vi "send command to printer.vi"(8 "error in (no error)":errorcluster, 10 "command to be sent":string, 11 "Domino Laser module Class in":refnum<class "Domino Laser module Class.lvclass">) -> (0 "error out":errorcluster, 1 "Command Excuted succeddfully?":bool, 2 "Recived message":string, 3 "Domino Laser module Class out":refnum<class "Domino Laser module Class.lvclass">)   [LabVIEW 2024, in "Domino LM.lvlib" / "Domino Laser module Class.lvclass"]
uses:
  CTRLS/Domino Laser module Class.lvclass
  CTRLS/Domino Laser module Class.lvclass/Domino Laser module Class.ctl
panel:
  out "sent":string[](array[string])
  out "Recived":string[](array[string])
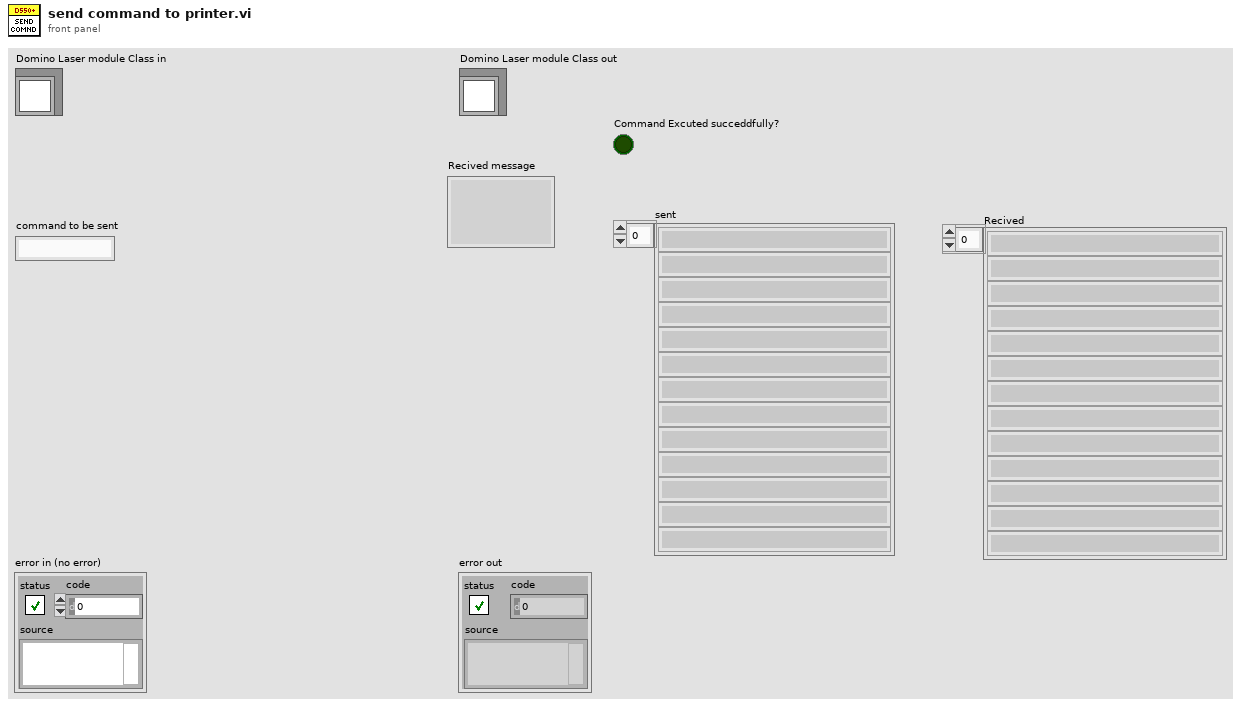
[diagram p1: front panel]
types:
  T1 = enum16{"Standard", "Buffered", "CRLF", "Immediate"}
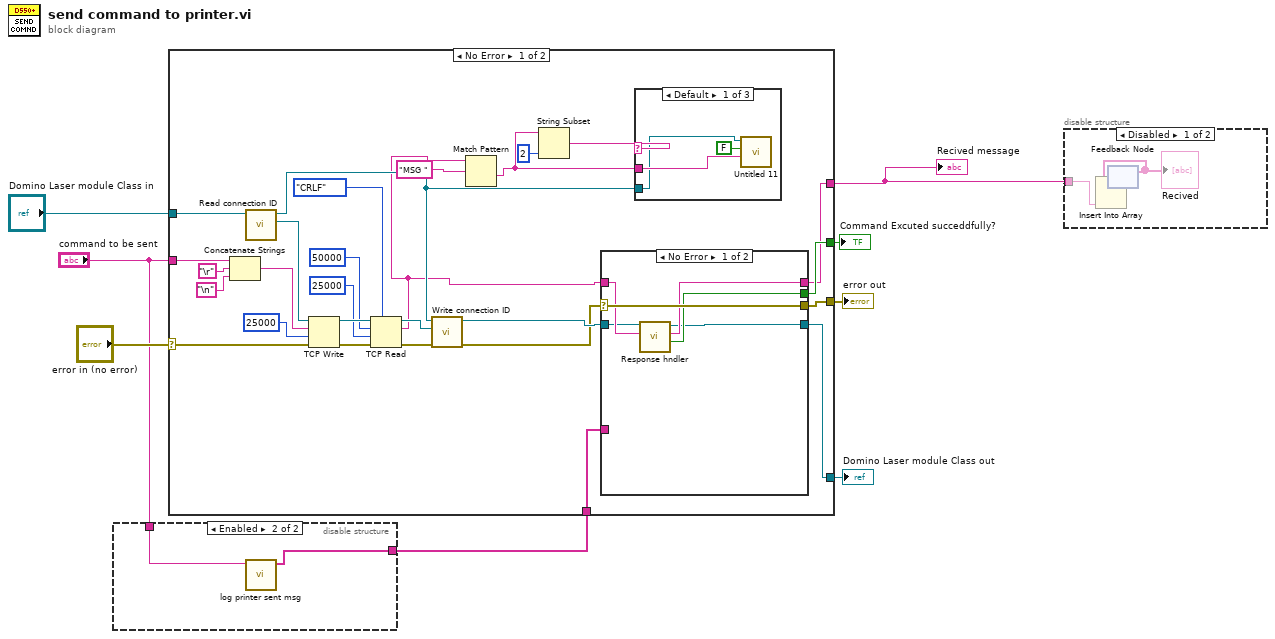
[diagram p0: block diagram]
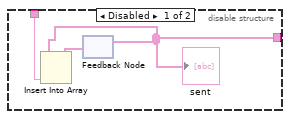
[diagram p3: hidden frame]
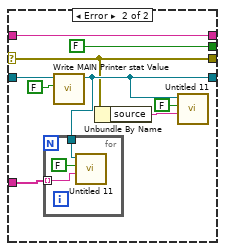
[diagram p4: hidden frame]
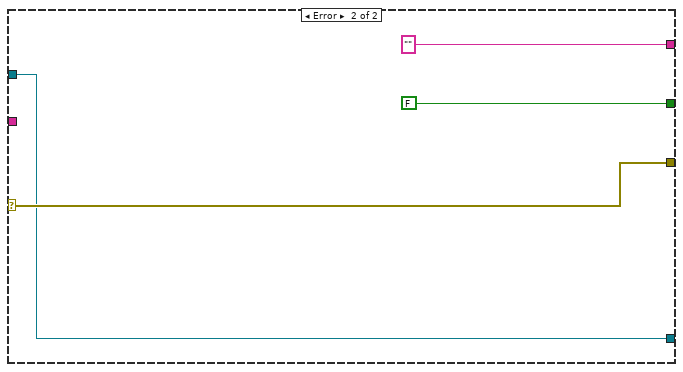
[diagram p7: hidden frame]
diagram:
  n1 = disable-structure shown="Enabled" {
    disable-tunnel: "command to be sent" -> [w10 w13]
    disable-tunnel: [w9 w12] -> w1
    frame Disabled {
      n2 = feedback #1() -> (w9:string[])  [unwired: 1 in]
      "sent" <- w9
      n3 = Insert Into Array(array=w9, new element=w10) -> (w11:string[])  [unwired: 1 in]
      n4 = feedback-in #1(w11) -> ()
    }
    frame Enabled {
      n5 = call "log printer sent msg.vi"("new element/subarray"=w13) -> ("sent 2"=w12:string[])  [unwired: 9 in, 1 out]
    }
  }
  n6 = case shown="No Error" "error in (no error)" {
    selector: "error in (no error)" -> [w28 w66]
    tunnel: [w17 w66] -> w7
    tunnel: [w16 w65] -> w5
    tunnel: "Domino Laser module Class in" -> [w27 w65]
    tunnel: [w15 "" ("data out")] -> w3
    tunnel: "command to be sent" -> [w29 _]
    tunnel: [w18 FALSE ("Command Excuted succeddfully?")] -> w4
    tunnel: w1 -> [w14 _]
    frame No Error {
      n7 = Concatenate Strings(w29, "\r", "\n") -> (w38:string)
      n8 = call "Read connection ID.vi"("Domino Laser module Class in"=w27) -> ("connection ID"=w39:refnum<k5>, "Domino Laser module Class out"=w22:refnum<class "Domino Laser module Class.lvclass">)  [unwired: 8 in, 1 out]
      n9 = TCP Write(connection ID=w39, data in=w38, error in (no error)=w28, 9:25000 ("timeout ms (25000)")) -> (connection ID out=w35:refnum<k5>, error out=w36:errorcluster)  [unwired: 1 out]
      n10 = TCP Read(connection ID=w35, bytes to read=50000 ("timeout ms (25000)"), error in (no error)=w36, 7:T1."CRLF" ("mode (standard)"), 9:25000 ("timeout ms (25000)")) -> (connection ID out=w33:refnum<k5>, data out=w19:string, error out=w32:errorcluster)
      n11 = call "Write connection ID.vi"("error in (no error)"=w32, "connection ID"=w33, "Domino Laser module Class in"=w22) -> ("error out"=w20:errorcluster, "Domino Laser module Class out"=w21:refnum<class "Domino Laser module Class.lvclass">)  [unwired: 7 in]
      n12 = Match Pattern(string=w19, regular expression="MSG ") -> (after substring=w25:string)  [unwired: 1 in, 3 out]
      n13 = String Subset(string=w25, length (rest)=2 ("length (rest)")) -> (substring=w23:string)  [unwired: 1 in]
      n14 = case shown="No Error" w20 {
        selector: w20 -> [w47 w51]
        tunnel: w21 -> [w43 w55]
        tunnel: [w42 w52] -> w16
        tunnel: w19 -> [w44 w54]
        tunnel: [w47 w51] -> w17
        tunnel: [w46 w54] -> w15
        tunnel: [w45 FALSE ("Command Excuted succeddfully?")] -> w18
        tunnel: w14 -> [_ w48]
        frame No Error {
          n15 = call "Response hndler.vi"("Recived MSG"=w44, "Domino LM.lvlib:Domino Laser module Class.lvclass"=w43) -> ("Command Excuted successfully?"=w45:bool, "printer response"=w46:string, "Domino LM.lvlib:Domino Laser module Class.lvclass 2"=w42:refnum<class "Domino Laser module Class.lvclass">)  [unwired: 7 in]
        }
        frame Error {
          n16 = call "Write MAIN Printer stat Value.vi"("Printer MIAN status"=FALSE ("Printer status"), "Domino Laser module Class in"=w55) -> ("Domino Laser module Class out"=w52:refnum<class "Domino Laser module Class.lvclass">)  [unwired: 8 in, 1 out]
          n17 = for {
            tunnel: w52 -> [w59]
            tunnel: w48 -> [w57] mode=indexing
            n18 = call "Untitled 11.vi"("MSG"=w57, "MSG Status"=FALSE, "Domino Laser module Class in"=w59) -> ()  [unwired: 7 in, 2 out]
          }
          n19 = Unbundle By Name(w51) -> ("source"=w50:string)
          n20 = call "Untitled 11.vi"("MSG"=w50, "MSG Status"=FALSE, "Domino Laser module Class in"=w52) -> ()  [unwired: 7 in, 2 out]
        }
      }
      n21 = case shown="Default" w23 {
        tunnel: w25 -> [w62 _ _]
        tunnel: w22 -> [w61 _ _]
        frame Default {
          n22 = call "Untitled 11.vi"("MSG"=w62, "MSG Status"=FALSE, "Domino Laser module Class in"=w61) -> ()  [unwired: 7 in, 2 out]
        }
        frame "25" {
        }
        frame "" {
        }
      }
    }
    frame Error {
    }
  }
  "error out" <- w7
  "Domino Laser module Class out" <- w5
  "Recived message" <- w3
  "Command Excuted succeddfully?" <- w4
  n23 = disable-structure shown="Disabled" {
    disable-tunnel: w3 -> [w69 _]
    frame Disabled {
      n24 = feedback #2() -> (w67:string[])  [unwired: 1 in]
      "Recived" <- w67
      n25 = Insert Into Array(array=w67, new element=w69) -> (w68:string[])  [unwired: 1 in]
      n26 = feedback-in #2(w68) -> ()
    }
    frame Enabled {
    }
  }
